vi "TimeoutTactic.vi"(6 "IndexInVector":dbl, 8 "error in (no error)":errorcluster, 9 "Game in":refnum<class "Game.lvclass">, 10 "Robot":refnum<class "Robot.lvclass">, 11 "TimeoutTactic in":refnum<class "TimeoutTactic.lvclass">) -> (0 "error out":errorcluster, 2 "Robot out":refnum<class "Robot.lvclass">, 3 "TimeoutTactic out":refnum<class "TimeoutTactic.lvclass">)   [LabVIEW 2018, in "TimeoutTactic.lvclass"]
uses:
  TimeoutTactic.lvclass
  C:/Users/nicolas.oliveira/roboime/SSL_AI/Tactic_class/Tactic.lvclass
  Robot_class/Robot.lvclass
  Game_class/Game.lvclass
  Tactic_class/Tactic.lvclass/Tactic.ctl
  Skillbook_class/Skillbook.lvclass/Skillbook.ctl
  TimeoutTactic.lvclass/TimeoutTactic.ctl
  Skillbook_class/Read TimeoutSkill.vi
  Tactic_class/Read Skillbook.vi
  Write States.vi
  Skillbook_class/Skillbook.lvclass
  TimeoutSkill_class/TimeoutSkill.lvclass
panel:
  out "x .or. y?":bool
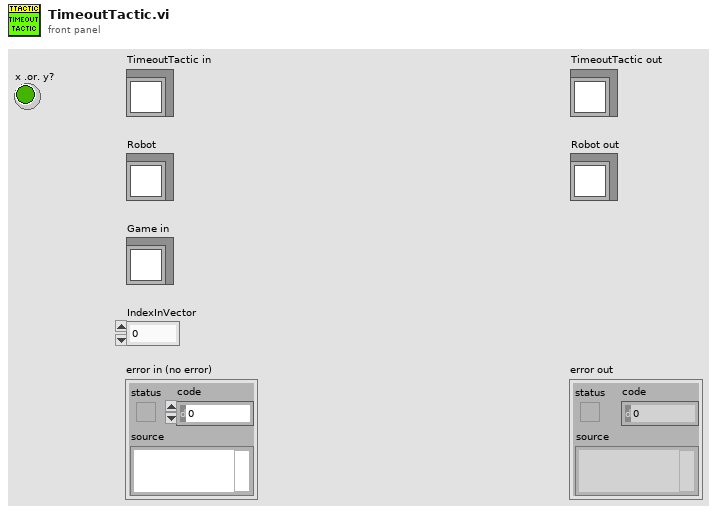
[diagram p1: front panel]
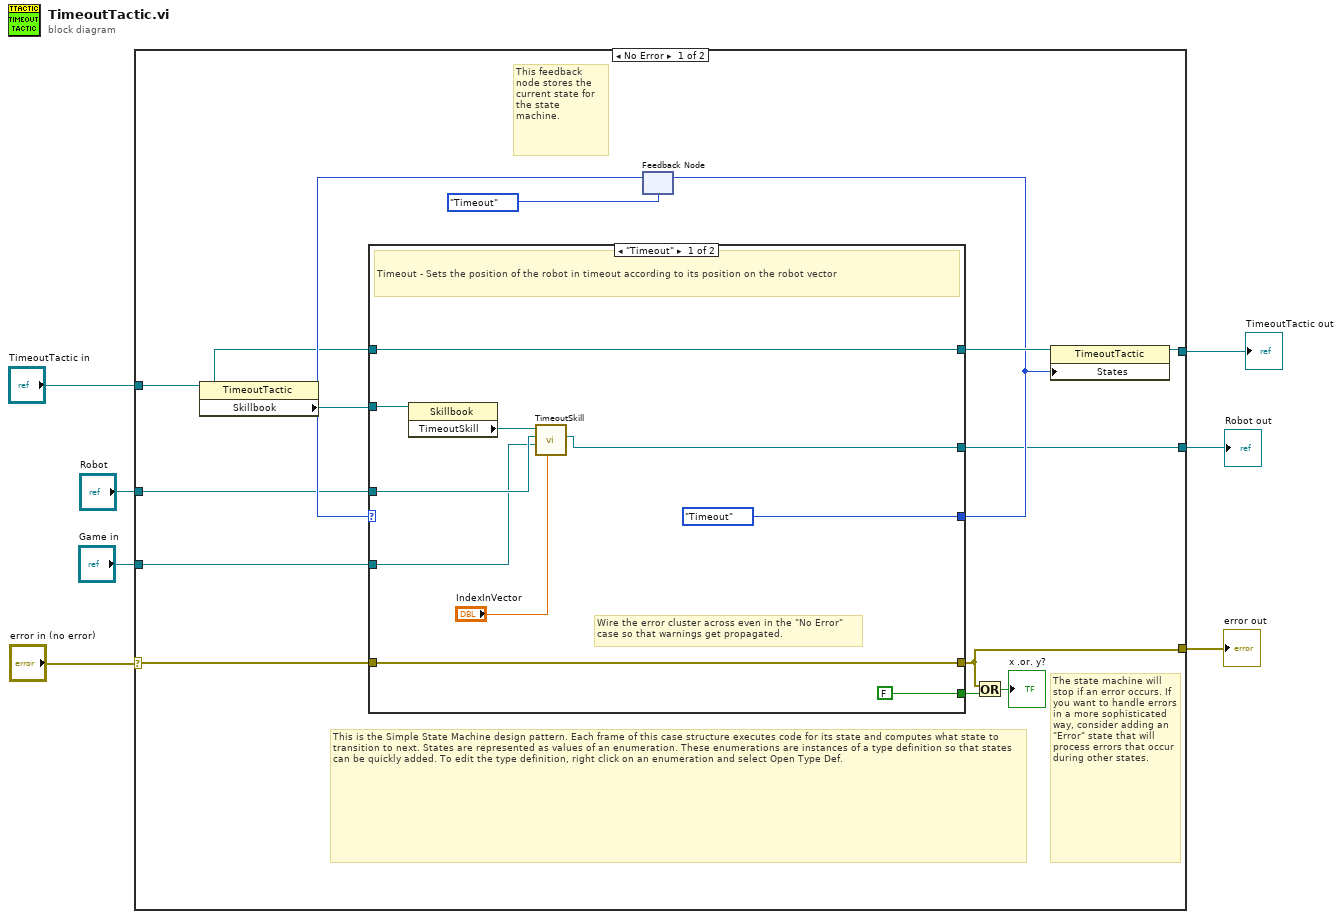
[diagram p0: block diagram]
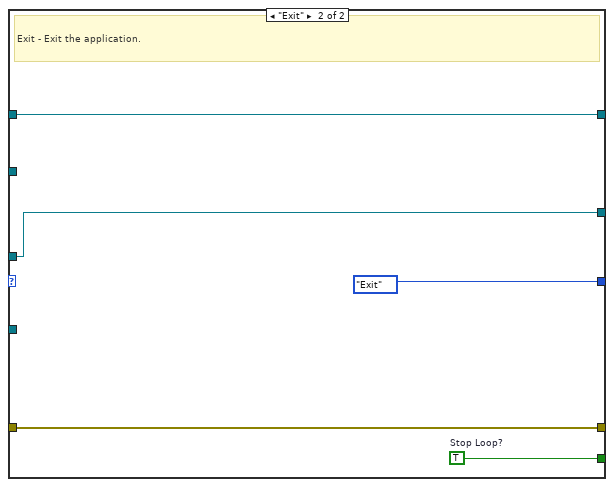
[diagram p2: hidden frame]
diagram:
  n1 = case shown="No Error" "error in (no error)" {
    selector: "error in (no error)" -> [w15 w39]
    tunnel: [w14 w39] -> w6
    tunnel: [w12 w38] -> w4
    tunnel: "TimeoutTactic in" -> [w13 w38]
    tunnel: "Game in" -> [w11 _]
    tunnel: "Robot" -> [w10 w37]
    tunnel: [w9 w37] -> w1
    frame No Error {
      # "The state machine will stop if an error occurs. If you want to handle errors in a more sophisticated way, consider adding an \"Error\" state that will process errors that occur during other states."
      # "This feedback node stores the current state for the state machine."
      # "This is the Simple State Machine design pattern. Each frame of this case structure executes code for its state and computes what state to transition to next. States are represented as values of an enumeration. These enumerations are instances of a type definition so that states can be quickly added. To edit the type definition, right click on an enumeration and select Open Type Def."
      # "Wire the error cluster across even in the \"No Error\"\ncase so that warnings get propagated."
      n2 = property class="TimeoutTactic"(reference=w13) -> ("Skillbook"=w18:refnum<class "Skillbook.lvclass">)  [unwired: 1 in, 2 out]
      n3 = feedback #1(enum16{"Exit", "Timeout"}."Timeout" ("States")) -> (w19:enum16{"Exit", "Timeout"})
      n4 = case shown="\"Timeout\"" w19 {
        tunnel: [enum16{"Exit", "Timeout"}."Timeout" ("States") enum16{"Exit", "Timeout"}."Exit" ("States")] -> w16
        tunnel: [FALSE ("Stop Loop?") w36] -> w21
        tunnel: w15 -> [w30 w35]
        tunnel: [w30 w35] -> w14
        tunnel: w18 -> [w29 _]
        tunnel: w10 -> [w26 w34]
        tunnel: [w25 w34] -> w9
        tunnel: [w28 w33] -> w17
        tunnel: w13 -> [w28 w33]
        tunnel: w11 -> [w24 _]
        frame "Timeout" {
          # "Timeout - Sets the position of the robot in timeout according to its position on the robot vector"
          n5 = property class="Skillbook"(reference=w29) -> ("TimeoutSkill"=w27:refnum<class "TimeoutSkill.lvclass">)  [unwired: 1 in, 2 out]
          n6 = call-dynamic "TimeoutSkill.vi"("IndexInVector"="IndexInVector", "Game"=w24, "Robot"=w26, "TimeoutSkill in"=w27) -> ("Robot out"=w25:refnum<class "Robot.lvclass">)  [unwired: 5 in, 2 out]
        }
        frame "Exit" {
          w36 = TRUE  # Stop Loop?
          # "Exit - Exit the application."
        }
      }
      n7 = feedback-in #1(w16) -> ()
      n8 = Or(x=w14, y=w21) -> (x .or. y?=→"x .or. y?":bool)
      n9 = property class="TimeoutTactic"(reference=w17, "States"=w16) -> (reference out=w12:refnum<class "TimeoutTactic.lvclass">)  [unwired: 1 in, 1 out]
    }
    frame Error {
    }
  }
  "error out" <- w6
  "TimeoutTactic out" <- w4
  "Robot out" <- w1
